vi "new http responder.vi"(8 "error in":errorcluster, 11 "http responder in":refnum<class "https responder.lvclass">) -> (0 "error out":errorcluster, 3 "http responder out":refnum<class "https responder.lvclass">)   [LabVIEW 2016, in "https responder.lvclass"]
uses:
  https responder.lvclass
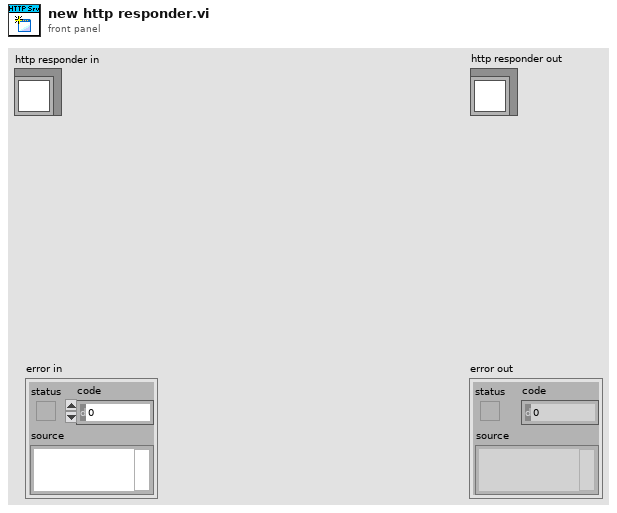
[diagram p1: front panel]
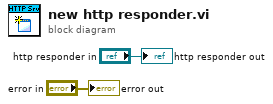
[diagram p0: block diagram]
diagram:
  "error out" <- "error in"
  "http responder out" <- "http responder in"
